vi "PicoScope5000aAdvancedTriggerSettingsV2.vi"(0 "error in":errorcluster, 1 "handle in":i16=16384, 3 "Trigger Conditions":T1 {"Digital Port 1" items=["Don't Care", "True", "False"]; "Digital Port 0" items=["Don't Care", "True", "False"]; "PWQ" items=["Don't Care", "True", "False"]; "Aux" items=["Don't Care", "True", "False"]; "Ext" items=["Don't Care", "True", "False"]; "Channel D" items=["Don't Care", "True", "False"]; "Channel C" items=["Don't Care", "True", "False"]; "Channel B" items=["Don't Care", "True", "False"]; "Channel A" items=["Don't Care", "True", "False"]; "Condition Logic" items=["AND", "OR", "XOR"]}, 4 "Trigger Delay":u32, 5 "Auto Trigger (us)":u64=1000000, 6 "Channel A Trigger Properties":T4={"thresholdUpper"=0, "thresholdUpperHysteresis"=0, "thresholdLower"=0, "thresholdLowerHysteresis"=0, "Threshold Mode"=0, "Direction"=2, "Available"=FALSE} {"Direction" items=["Above / Inside", "Below / Outside", "Rising / Enter", "Falling / Exit", "Rising or Falling / Enter or Exit", "Above Lower", "Below Lower", "Rising Lower", "Falling Lower", "Positive Runt", "Negative Runt"]; "Threshold Mode" items=["Level", "Window"]}, 7 "Channel D Trigger Properties":T4={"thresholdUpper"=0, "thresholdUpperHysteresis"=0, "thresholdLower"=0, "thresholdLowerHysteresis"=0, "Threshold Mode"=0, "Direction"=2, "Available"=FALSE} {"Direction" items=["Above / Inside", "Below / Outside", "Rising / Enter", "Falling / Exit", "Rising or Falling / Enter or Exit", "Above Lower", "Below Lower", "Rising Lower", "Falling Lower", "Positive Runt", "Negative Runt"]; "Threshold Mode" items=["Level", "Window"]}, 8 "Channel B Trigger Properties":T4={"thresholdUpper"=0, "thresholdUpperHysteresis"=0, "thresholdLower"=0, "thresholdLowerHysteresis"=0, "Threshold Mode"=0, "Direction"=2, "Available"=FALSE} {"Direction" items=["Above / Inside", "Below / Outside", "Rising / Enter", "Falling / Exit", "Rising or Falling / Enter or Exit", "Above Lower", "Below Lower", "Rising Lower", "Falling Lower", "Positive Runt", "Negative Runt"]; "Threshold Mode" items=["Level", "Window"]}, 10 "Digital Port  0":T3 {"Direction Channel 7" items=["Don't Care", "Low", "High", "Rising", "Falling"]; "Direction Channel 6" items=["Don't Care", "Low", "High", "Rising", "Falling"]; "Direction Channel 5" items=["Don't Care", "Low", "High", "Rising", "Falling"]; "Direction Channel 4" items=["Don't Care", "Low", "High", "Rising", "Falling"]; "Direction Channel 3" items=["Don't Care", "Low", "High", "Rising", "Falling"]; "Direction Channel 2" items=["Don't Care", "Low", "High", "Rising", "Falling"]; "Direction Channel 1" items=["Don't Care", "Low", "High", "Rising", "Falling"]; "Direction Channel 0" items=["Don't Care", "Low", "High", "Rising", "Falling"]}, 11 "Ext. Trigger Properties":T4={"thresholdUpper"=0, "thresholdUpperHysteresis"=0, "thresholdLower"=0, "thresholdLowerHysteresis"=0, "Threshold Mode"=0, "Direction"=2, "Available"=FALSE} {"Direction" items=["Above / Inside", "Below / Outside", "Rising / Enter", "Falling / Exit", "Rising or Falling / Enter or Exit", "Above Lower", "Below Lower", "Rising Lower", "Falling Lower", "Positive Runt", "Negative Runt"]; "Threshold Mode" items=["Level", "Window"]}, 12 "Digital Port  1":T2 {"Direction Channel 15" items=["Don't Care", "Low", "High", "Rising", "Falling"]; "Direction Channel 14" items=["Don't Care", "Low", "High", "Rising", "Falling"]; "Direction Channel 13" items=["Don't Care", "Low", "High", "Rising", "Falling"]; "Direction Channel 12" items=["Don't Care", "Low", "High", "Rising", "Falling"]; "Direction Channel 11" items=["Don't Care", "Low", "High", "Rising", "Falling"]; "Direction Channel 10" items=["Don't Care", "Low", "High", "Rising", "Falling"]; "Direction Channel 9" items=["Don't Care", "Low", "High", "Rising", "Falling"]; "Direction Channel 8" items=["Don't Care", "Low", "High", "Rising", "Falling"]}, 13 "Aux. Trigger Properties (DO NOT USE)":T4={"thresholdUpper"=0, "thresholdUpperHysteresis"=0, "thresholdLower"=0, "thresholdLowerHysteresis"=0, "Threshold Mode"=0, "Direction"=2, "Available"=FALSE} {"Direction" items=["Above / Inside", "Below / Outside", "Rising / Enter", "Falling / Exit", "Rising or Falling / Enter or Exit", "Above Lower", "Below Lower", "Rising Lower", "Falling Lower", "Positive Runt", "Negative Runt"]; "Threshold Mode" items=["Level", "Window"]}, 16 "Channel C Trigger Properties":T4={"thresholdUpper"=0, "thresholdUpperHysteresis"=0, "thresholdLower"=0, "thresholdLowerHysteresis"=0, "Threshold Mode"=0, "Direction"=2, "Available"=FALSE} {"Direction" items=["Above / Inside", "Below / Outside", "Rising / Enter", "Falling / Exit", "Rising or Falling / Enter or Exit", "Above Lower", "Below Lower", "Rising Lower", "Falling Lower", "Positive Runt", "Negative Runt"]; "Threshold Mode" items=["Level", "Window"]}, 18 "Pulse Width Qualifier Conditions":T6 {"Condition Logic" items=["AND", "OR", "XOR"]}, 19 "Pulse Width Qualifier Settings":T5={"Direction"=2, "Lower Limit"=0, "Upper Limit"=0, "Pulse Width Type"=0} {"Pulse Width Type" items=["None", "Less Than", "Greater Than", "In Range", "Out of Range"]; "Direction" items=["Rising"=2, "Falling"=3, "Rising Lower"=7, "Above"=0, "Below"=1, "Rising or Falling"=4, "Falling Lower"=8, "Below Lower"=6, "Above Lower"=5]}) -> (14 "error out":errorcluster, 15 "handle out":i16=16384)   [LabVIEW 2010]
doc: "This VI is an interface for the advanced trigger features of the oscilloscope (Using V2 functions now recommended)\nA simple trigger can be set using PicoScope5000aSettings.vi, in which case it is not necessary to use this VI."
uses:
  ps5000a.dll
panel:
  out "XOR Debug Array":u32[][](array[numeric])
  in  "SetTrigger Info Action XOR":bool=TRUE
  in  "SetTrigger Info Action OR":bool=TRUE
  # "For Condition Logic Suggested settings;\nFor AND, XOR logic-(parallel triggers)\nUse level-type triggers (Level or Inside/outside Window Triggers)\n\nFor OR logic- (single channel)\nUse edge types (e.g. rising, falling, entering window)"
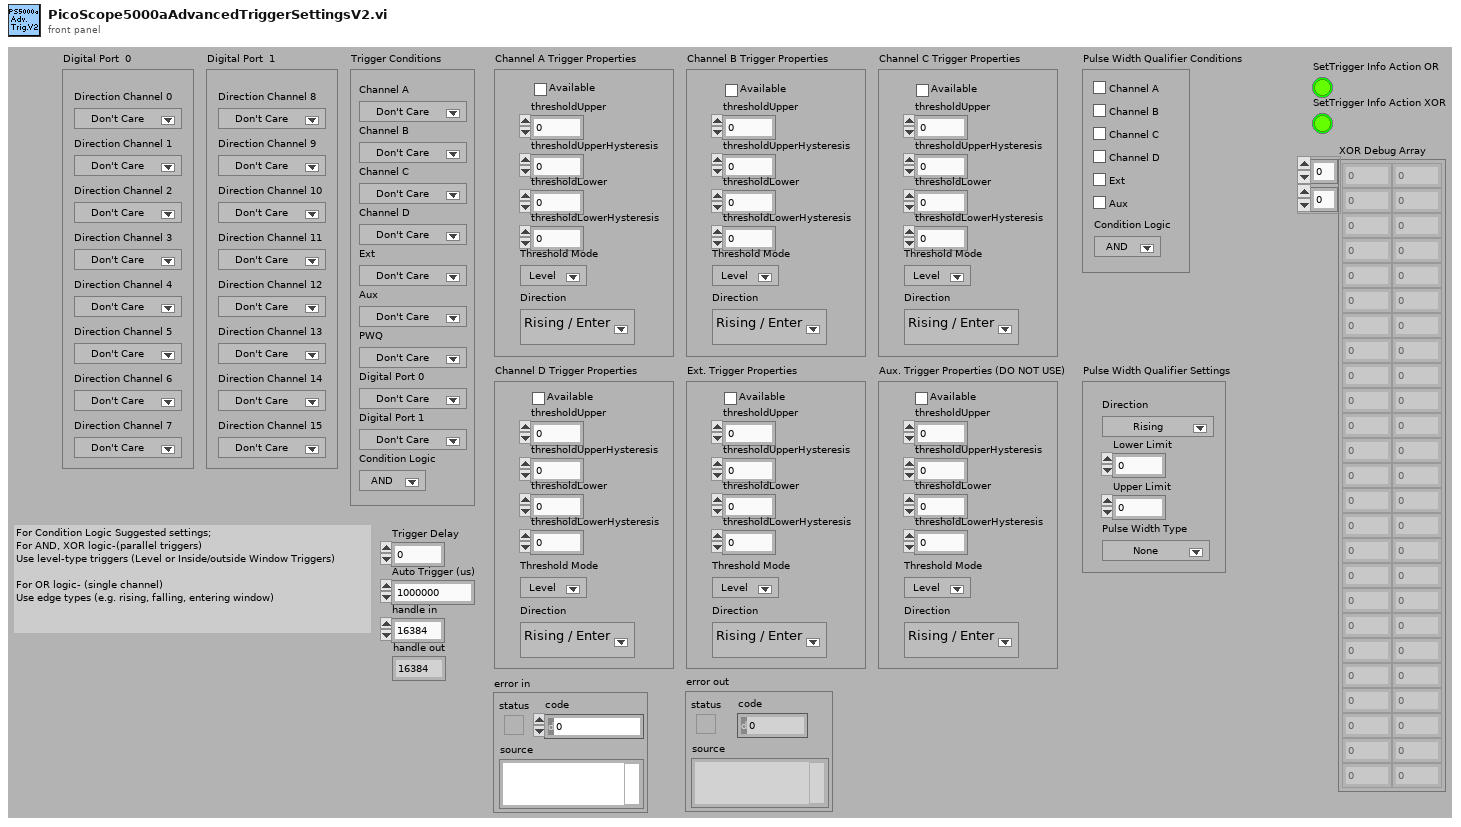
[diagram p1: front panel]
types:
  T1 = cluster{"Channel A":u16, "Channel B":u16, "Channel C":u16, "Channel D":u16, "Ext":u16, "Aux":u16, "PWQ":u16, "Digital Port 0":u16, "Digital Port 1":u16, "Condition Logic":u16}
  T2 = cluster{"Direction Channel 8":u16, "Direction Channel 9":u16, "Direction Channel 10":u16, "Direction Channel 11":u16, "Direction Channel 12":u16, "Direction Channel 13":u16, "Direction Channel 14":u16, "Direction Channel 15":u16}
  T3 = cluster{"Direction Channel 0":u16, "Direction Channel 1":u16, "Direction Channel 2":u16, "Direction Channel 3":u16, "Direction Channel 4":u16, "Direction Channel 5":u16, "Direction Channel 6":u16, "Direction Channel 7":u16}
  T4 = cluster{"thresholdUpper":i16, "thresholdUpperHysteresis":u16, "thresholdLower":i16, "thresholdLowerHysteresis":u16, "Threshold Mode":i32, "Direction":i32, "Available":bool}
  T5 = cluster{"Direction":u32, "Lower Limit":u32, "Upper Limit":u32, "Pulse Width Type":u32}
  T6 = cluster{"Channel A":bool, "Channel B":bool, "Channel C":bool, "Channel D":bool, "Aux":bool, "Condition Logic":u16, "Ext":bool}
  T7 = cluster{"status":bool, "code":u32, "source":string}
  T8 = cluster{"thresholdUpper":i16, "thresholdUpperHysteresis":u16, "thresholdLower":i16, "thresholdLowerHysteresis":u16, "Threshold Mode":i32, "Direction":i32, "Available":bool}[]
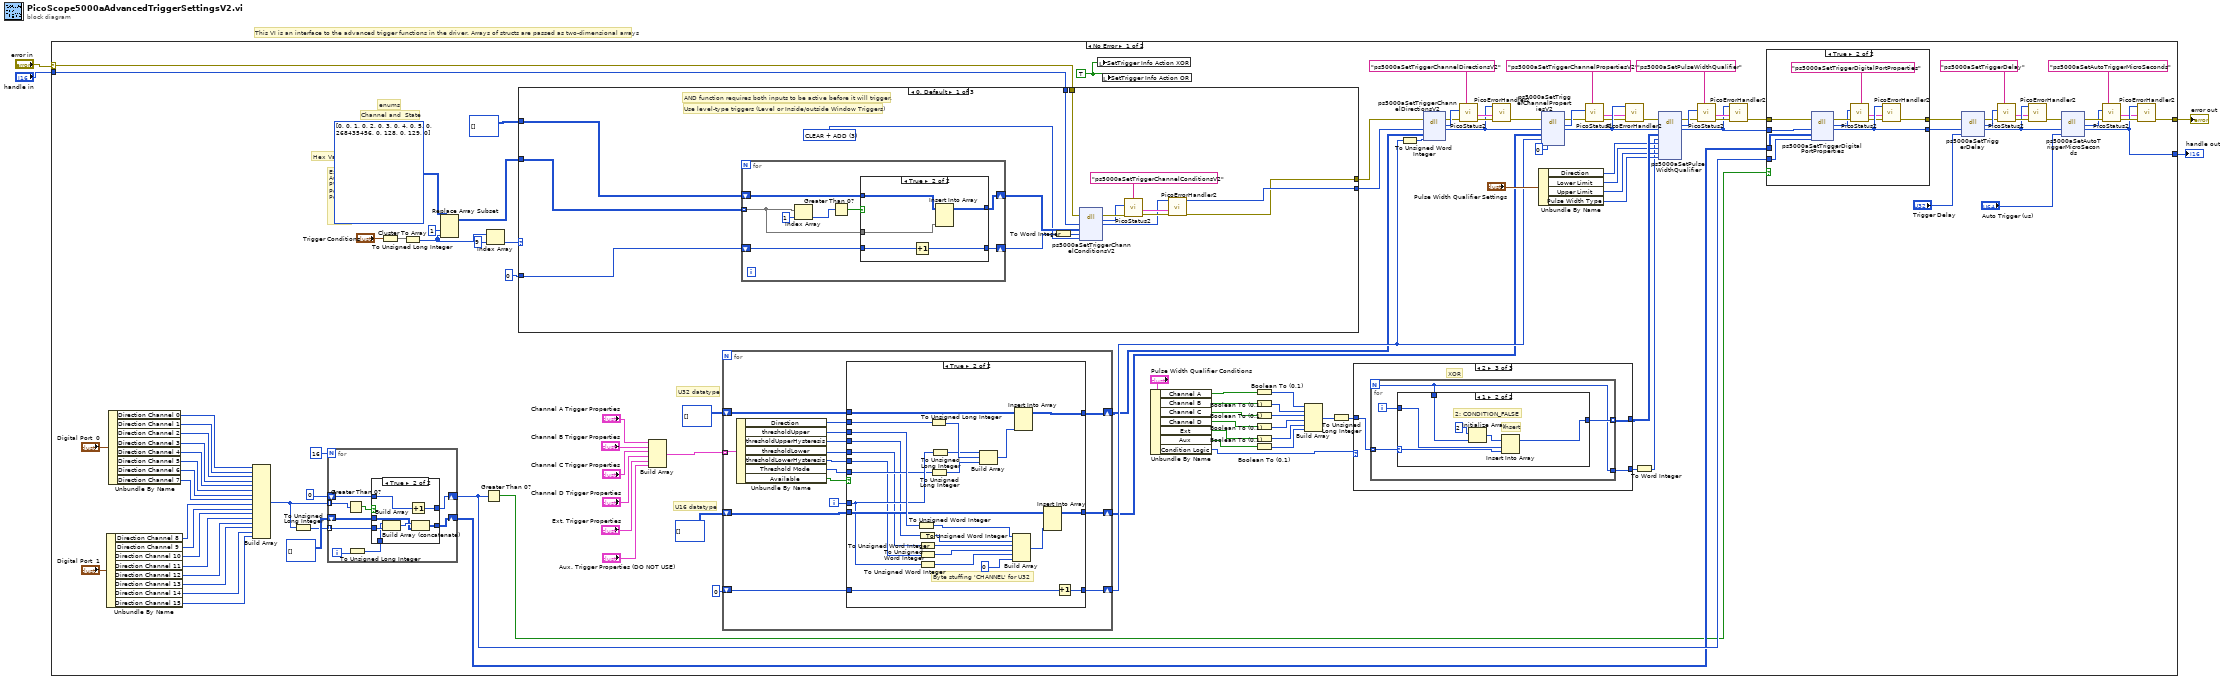
[diagram p0: block diagram]
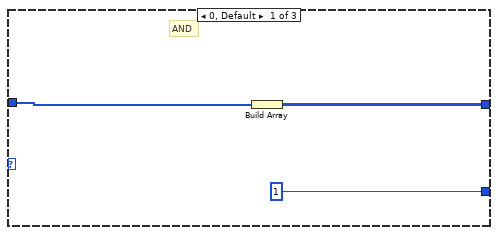
[diagram p4: hidden frame]
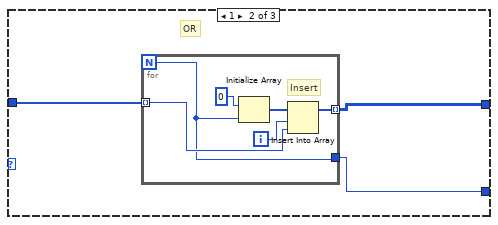
[diagram p5: hidden frame]
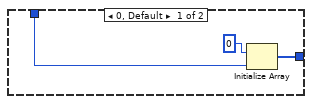
[diagram p6: hidden frame]
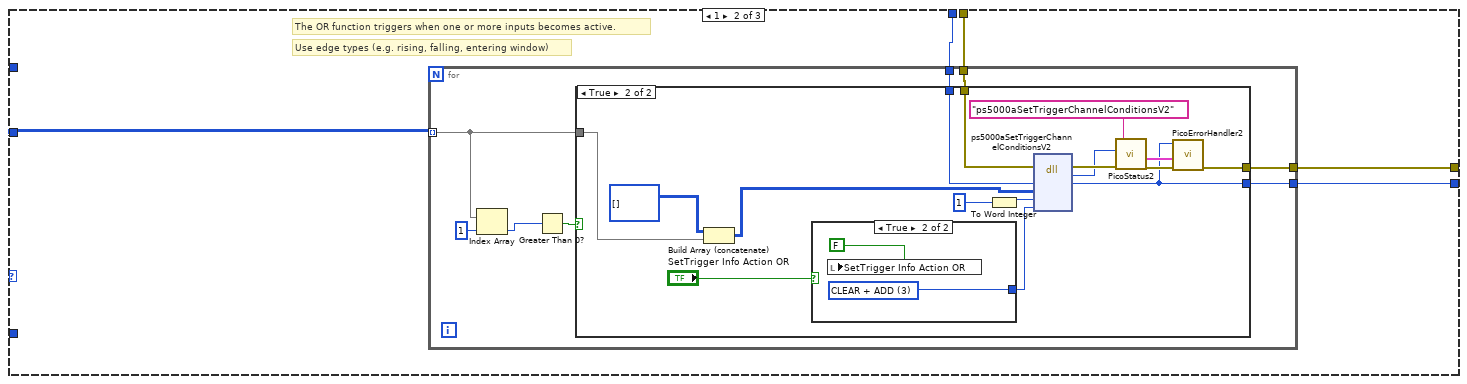
[diagram p9: hidden frame]
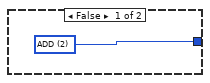
[diagram p11: hidden frame]
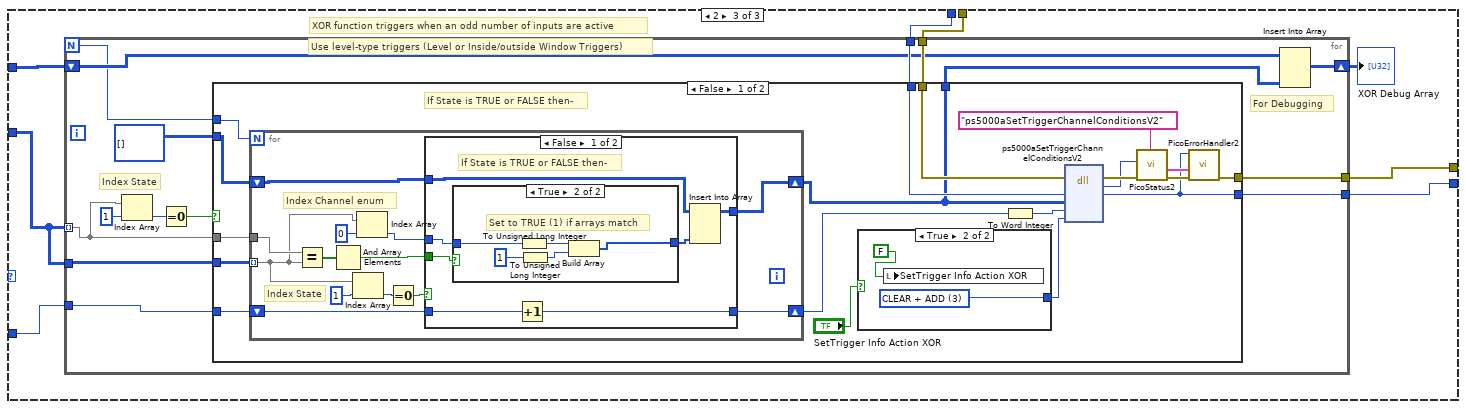
[diagram p12: hidden frame]
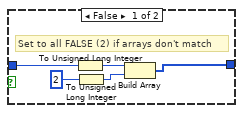
[diagram p13: hidden frame]
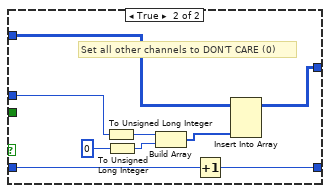
[diagram p14: hidden frame]
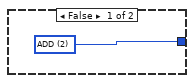
[diagram p15: hidden frame]
diagram:
  # "This VI is an interface to the advanced trigger functions in the driver. Arrays of structs are passed as two-dimensional arrays"
  n1 = case shown="No Error" "error in" {
    selector: "error in" -> [w60 w377]
    tunnel: "handle in" -> [w59 w378]
    tunnel: [w47 w378] -> w2
    tunnel: [w48 w377] -> w1
    frame No Error {
      w53 = TRUE ("Boolean")
      # "enums"
      # "Ext\nAux\nPWQ\nPort0\nPort1"
      # "Channel and  State"
      # "Hex Values"
      # "U16 datatype"
      # "U32 datatype"
      n2 = Unbundle By Name("Digital Port  1") -> ("Direction Channel 8"=w83:u16, "Direction Channel 9"=w82:u16, "Direction Channel 10"=w81:u16, "Direction Channel 11"=w80:u16, "Direction Channel 12"=w79:u16, "Direction Channel 13"=w78:u16, "Direction Channel 14"=w77:u16, "Direction Channel 15"=w76:u16)
      n3 = Unbundle By Name("Digital Port  0") -> ("Direction Channel 0"=w75:u16, "Direction Channel 1"=w92:u16, "Direction Channel 2"=w91:u16, "Direction Channel 3"=w90:u16, "Direction Channel 4"=w89:u16, "Direction Channel 5"=w88:u16, "Direction Channel 6"=w87:u16, "Direction Channel 7"=w86:u16)
      n4 = Build Array(w75, w92, w91, w90, w89, w88, w87, w86, w83, w82, w81, w80, w79, w78, w77, w76) -> (w66:u16[])
      n5 = To Unsigned Long Integer(number=w66) -> (unsigned 32bit integer=w67:u32[])
      n6 = for {
        N: 16 -> [_]
        tunnel: w67 -> [w143] mode=indexing
        shift-right: [w144] -> w71
        shift-left: i16 0 -> [w145]
        shift-right: [w141] -> w70
        shift-left: u32[][] [] -> [w142]
        tunnel: w66 -> [w139] mode=indexing
        i -> [w138]
        n7 = Greater Than 0?(x=w139) -> (x > 0?=w140:bool)
        n8 = To Unsigned Long Integer(number=w138) -> (unsigned 32bit integer=w137:u32)
        n9 = case shown="True" w140 {
          tunnel: w145 -> [w147 w154]
          tunnel: [w147 w151] -> w144
          tunnel: w143 -> [_ w153]
          tunnel: w137 -> [_ w152]
          tunnel: w142 -> [w146 w149]
          tunnel: [w146 w148] -> w141
          frame False {
          }
          frame True {
            n10 = Build Array(w152, w153) -> (w150:u32[])
            n11 = Increment(x=w154) -> (x+1=w151:i16)
            n12 = Build Array (concatenate)(w150, w149) -> (w148:u32[][])
          }
        }
      }
      n13 = Cluster To Array(cluster="Trigger Conditions") -> (array=w42:u16[])
      n14 = To Unsigned Long Integer(number=w42) -> (unsigned 32bit integer=w40:u32[])
      n15 = Replace Array Subset(array=u32[][] [[0, 0], [1, 0], [2, 0], [3, 0], [4, 0], [5, 0], [268435456, 0], [128, 0], [129, 0]], new element=w40, index (col)=1 ("disabled index (col)")) -> (w41:u32[][])  [unwired: 1 in]
      n16 = Greater Than 0?(x=w71) -> (x > 0?=w46:bool)
      n17 = Index Array(array=w40, index=9) -> (element=w38:u32)
      n18 = case shown="0, Default" w38 {
        tunnel: u32[][] [] -> [w240 _ w293]
        tunnel: i16 0 -> [w239 _ w290]
        tunnel: w60 -> [w233 w260 w297]
        tunnel: w59 -> [w232 w259 w296]
        tunnel: [w225 w258 w295] -> w58
        tunnel: [w226 w257 w294] -> w57
        tunnel: w41 -> [w229 w256 w291]
        frame 0, Default {
          w230 = u32 3 items=["CLEAR + ADD"=3, "CLEAR"=1, "ADD"=2] ("Condition Action")
          # "AND function requires both inputs to be active before it will trigger."
          # "Use level-type triggers (Level or Inside/outside Window Triggers)"
          n19 = for {
            shift-right: [w247] -> w235
            shift-left: w239 -> [w246]
            shift-right: [w245] -> w231
            shift-left: w240 -> [w248]
            tunnel: w229 -> [w243] mode=indexing
            n20 = Index Array(array=w243, index=1) -> (element=w242:u32)
            n21 = Greater Than 0?(x=w242) -> (x > 0?=w244:bool)
            n22 = case shown="True" w244 {
              tunnel: w248 -> [w250 w255]
              tunnel: [w250 w254] -> w245
              tunnel: [w249 w253] -> w247
              tunnel: w246 -> [w249 w252]
              tunnel: w243 -> [_ w251]
              frame False {
              }
              frame True {
                n23 = Increment(x=w252) -> (x+1=w253:i16)
                n24 = Insert Into Array(array=w255, new element=w251) -> (w254:u32[][])  [unwired: 2 in]
              }
            }
          }
          n25 = To Word Integer(number=w235) -> (16bit integer=w238:i16)
          n26 = dll-call lib="ps5000a.dll" fn="ps5000aSetTriggerChannelConditionsV2" ("ps3000.dll:_ps3000_open_unit@0")(error in=w233, "handle"=w232, "conditions"=w231, "nConditions"=w238, "info"=w230) -> (error out=w237:errorcluster, "PICO_STATUS"=w236:u32, "handle"=w226:i16)  [unwired: 5 in, 1 out]
          n27 = call "PicoStatus2.vi"("PICO source"="ps5000aSetTriggerChannelConditionsV2" ("source"), "Error in"=w237, "PICO STATUS"=w236) -> ("error out"=w228:errorcluster, "PICO_STATUS out"=w227:T7)  [unwired: 5 in]
          n28 = call "PicoErrorHandler2.vi"("error in (no error)"=w228, "PICO_STATUS in"=w227, "handle In"=w226) -> ("error out"=w225:errorcluster)  [unwired: 8 in]
        }
        frame 1 {
          # "Use edge types (e.g. rising, falling, entering window)"
          # "The OR function triggers when one or more inputs becomes active."
          n29 = for {
            tunnel: w260 -> [w268]
            tunnel: w259 -> [w267]
            tunnel: [w266] -> w258
            tunnel: [w265] -> w257
            tunnel: w256 -> [w263] mode=indexing
            n30 = Index Array(array=w263, index=1) -> (element=w262:u32)
            n31 = Greater Than 0?(x=w262) -> (x > 0?=w261:bool)
            n32 = case shown="True" w261 {
              tunnel: w268 -> [w269 w282]
              tunnel: w267 -> [w270 w281]
              tunnel: [w269 w271] -> w266
              tunnel: [w270 w272] -> w265
              tunnel: w263 -> [_ w275]
              frame False {
              }
              frame True {
                n33 = Build Array (concatenate)(u32[][] [], w275) -> (w277:u32[][])
                n34 = case shown="True" "SetTrigger Info Action OR" {
                  tunnel: [w287 w289] -> w280
                  frame False {
                    w287 = u32 2 items=["CLEAR"=1, "ADD"=2, "CLEAR + ADD"=3] ("Condition Action")
                  }
                  frame True {
                    w289 = u32 3 items=["CLEAR"=1, "ADD"=2, "CLEAR + ADD"=3] ("Condition Action")
                    n35 = local write "SetTrigger Info Action OR"(FALSE ("Boolean")) -> ()
                  }
                }
                n36 = To Word Integer(number=i16 1) -> (16bit integer=w286:i16)
                n37 = dll-call lib="ps5000a.dll" fn="ps5000aSetTriggerChannelConditionsV2" ("ps3000.dll:_ps3000_open_unit@0")(error in=w282, "handle"=w281, "conditions"=w277, "nConditions"=w286, "info"=w280) -> (error out=w285:errorcluster, "PICO_STATUS"=w284:u32, "handle"=w272:i16)  [unwired: 5 in, 1 out]
                n38 = call "PicoStatus2.vi"("PICO source"="ps5000aSetTriggerChannelConditionsV2" ("source"), "Error in"=w285, "PICO STATUS"=w284) -> ("error out"=w274:errorcluster, "PICO_STATUS out"=w273:T7)  [unwired: 5 in]
                n39 = call "PicoErrorHandler2.vi"("error in (no error)"=w274, "PICO_STATUS in"=w273, "handle In"=w272) -> ("error out"=w271:errorcluster)  [unwired: 8 in]
              }
            }
          }
        }
        frame 2 {
          # "Use level-type triggers (Level or Inside/outside Window Triggers)"
          # "XOR function triggers when an odd number of inputs are active"
          n40 = for {
            N -> [w305]
            tunnel: w297 -> [w312]
            tunnel: w296 -> [w311]
            tunnel: [w310] -> w295
            tunnel: [w309] -> w294
            shift-right: [w307] -> w292
            shift-left: w293 -> [w308]
            tunnel: w291 -> [w299] mode=indexing
            tunnel: w291 -> [w302]
            tunnel: w290 -> [w303]
            # "Index State"
            # "For Debugging"
            n41 = Index Array(array=w299, index=1) -> (element=w300:u32)
            n42 = Equal To 0?(x=w300) -> (x = 0?=w298:bool)
            n43 = case shown="False" w298 {
              tunnel: w312 -> [w331 w374]
              tunnel: w311 -> [w330 w375]
              tunnel: [w316 w374] -> w310
              tunnel: [w313 w375] -> w309
              tunnel: [w328 w376] -> w306
              tunnel: w305 -> [w327 _]
              tunnel: u32[][] [] -> [w326 w376]
              tunnel: w303 -> [w325 _]
              tunnel: w302 -> [w324 _]
              tunnel: w299 -> [w323 _]
              frame False {
                # "If State is TRUE or FALSE then-"
                n44 = for {
                  N: w327 -> [_]
                  shift-right: [w343] -> w329
                  shift-left: w325 -> [w344]
                  shift-right: [w332] -> w328
                  shift-left: w326 -> [w333]
                  tunnel: w323 -> [w340]
                  tunnel: w324 -> [w336] mode=indexing
                  # "Index State"
                  # "Index Channel enum"
                  n45 = Equal?(x=w340, y=w336) -> (x = y?=w334:bool[])
                  n46 = And Array Elements(Boolean array=w334) -> (logical AND=w339:bool)
                  n47 = Index Array(array=w336, index=1) -> (element=w337:u32)
                  n48 = Index Array(array=w336, index=0) -> (element=w341:u32)
                  n49 = Equal To 0?(x=w337) -> (x = 0?=w335:bool)
                  n50 = case shown="False" w335 {
                    tunnel: w344 -> [w351 w362]
                    tunnel: [w350 w363] -> w343
                    tunnel: w341 -> [w349 w366]
                    tunnel: w339 -> [w348 _]
                    tunnel: w333 -> [w347 w365]
                    tunnel: [w345 w364] -> w332
                    frame False {
                      # "If State is TRUE or FALSE then-"
                      n51 = case shown="True" w348 {
                        tunnel: [w356 w361] -> w346
                        tunnel: w349 -> [w355 w360]
                        frame False {
                          # "Set to all FALSE (2) if arrays don't match"
                          n52 = To Unsigned Long Integer(number=w355) -> (unsigned 32bit integer=w353:u32)
                          n53 = To Unsigned Long Integer(number=u32 2) -> (unsigned 32bit integer=w354:u32)
                          n54 = Build Array(w353, w354) -> (w356:u32[])
                        }
                        frame True {
                          # "Set to TRUE (1) if arrays match"
                          n55 = To Unsigned Long Integer(number=w360) -> (unsigned 32bit integer=w358:u32)
                          n56 = To Unsigned Long Integer(number=u32 1) -> (unsigned 32bit integer=w359:u32)
                          n57 = Build Array(w358, w359) -> (w361:u32[])
                        }
                      }
                      n58 = Increment(x=w351) -> (x+1=w350:i16)
                      n59 = Insert Into Array(array=w347, new element=w346) -> (w345:u32[][])  [unwired: 2 in]
                    }
                    frame True {
                      # "Set all other channels to DON'T CARE (0)"
                      n60 = To Unsigned Long Integer(number=w366) -> (unsigned 32bit integer=w368:u32)
                      n61 = To Unsigned Long Integer(number=u32 0) -> (unsigned 32bit integer=w369:u32)
                      n62 = Build Array(w368, w369) -> (w370:u32[])
                      n63 = Increment(x=w362) -> (x+1=w363:i16)
                      n64 = Insert Into Array(array=w365, new element=w370) -> (w364:u32[][])  [unwired: 2 in]
                    }
                  }
                }
                n65 = case shown="True" "SetTrigger Info Action XOR" {
                  tunnel: [w371 w373] -> w318
                  frame False {
                    w371 = u32 2 items=["CLEAR + ADD"=3, "CLEAR"=1, "ADD"=2] ("Condition Action")
                  }
                  frame True {
                    w373 = u32 3 items=["CLEAR + ADD"=3, "CLEAR"=1, "ADD"=2] ("Condition Action")
                    n66 = local write "SetTrigger Info Action XOR"(FALSE ("Boolean")) -> ()
                  }
                }
                n67 = To Word Integer(number=w329) -> (16bit integer=w322:i16)
                n68 = dll-call lib="ps5000a.dll" fn="ps5000aSetTriggerChannelConditionsV2" ("ps3000.dll:_ps3000_open_unit@0")(error in=w331, "handle"=w330, "conditions"=w328, "nConditions"=w322, "info"=w318) -> (error out=w321:errorcluster, "PICO_STATUS"=w317:u32, "handle"=w313:i16)  [unwired: 5 in, 1 out]
                n69 = call "PicoStatus2.vi"("PICO source"="ps5000aSetTriggerChannelConditionsV2" ("source"), "Error in"=w321, "PICO STATUS"=w317) -> ("error out"=w315:errorcluster, "PICO_STATUS out"=w314:T7)  [unwired: 5 in]
                n70 = call "PicoErrorHandler2.vi"("error in (no error)"=w315, "PICO_STATUS in"=w314, "handle In"=w313) -> ("error out"=w316:errorcluster)  [unwired: 8 in]
              }
              frame True {
              }
            }
            n71 = Insert Into Array(array=w308, new element=w306) -> (w307:u32[][])  [unwired: 2 in]
          }
          "XOR Debug Array" <- w292
        }
      }
      n72 = Build Array("Channel A Trigger Properties", "Channel B Trigger Properties", "Channel C Trigger Properties", "Channel D Trigger Properties", "Ext. Trigger Properties", "Aux. Trigger Properties (DO NOT USE)") -> (w121:T8)
      n73 = for {
        tunnel: w121 -> [w192] mode=indexing
        shift-right: [w189] -> w63
        shift-left: i16 0 -> [w188]
        shift-right: [w186] -> w36
        shift-left: u16[][] [] -> [w187]
        shift-right: [w185] -> w37
        shift-left: u32[][] [] -> [w184]
        i -> [w190]
        n74 = Unbundle By Name(w192) -> ("Direction"=w183:i32, "thresholdUpper"=w197:i16, "thresholdUpperHysteresis"=w196:u16, "thresholdLower"=w195:i16, "thresholdLowerHysteresis"=w194:u16, "Threshold Mode"=w193:i32, "Available"=w191:bool)
        n75 = case shown="True" w191 {
          tunnel: w197 -> [_ w224]
          tunnel: w196 -> [_ w204]
          tunnel: w195 -> [_ w203]
          tunnel: w194 -> [_ w202]
          tunnel: w193 -> [_ w212]
          tunnel: w190 -> [_ w214]
          tunnel: [w200 w222] -> w189
          tunnel: w188 -> [w200 w221]
          tunnel: [w199 w219] -> w186
          tunnel: w187 -> [w199 w218]
          tunnel: [w198 w217] -> w185
          tunnel: w184 -> [w198 w216]
          tunnel: w183 -> [_ w213]
          frame False {
          }
          frame True {
            # "Byte stuffing 'CHANNEL' for U32"
            n76 = To Unsigned Word Integer(number=w224) -> (unsigned 16bit integer=w206:u16)
            n77 = To Unsigned Word Integer(number=w204) -> (unsigned 16bit integer=w205:u16)
            n78 = To Unsigned Word Integer(number=w203) -> (unsigned 16bit integer=w201:u16)
            n79 = To Unsigned Word Integer(number=w202) -> (unsigned 16bit integer=w207:u16)
            n80 = To Unsigned Word Integer(number=w214) -> (unsigned 16bit integer=w208:u16)
            n81 = To Unsigned Long Integer(number=w213) -> (unsigned 32bit integer=w210:u32)
            n82 = To Unsigned Long Integer(number=w212) -> (unsigned 32bit integer=w211:u32)
            n83 = To Unsigned Long Integer(number=w214) -> (unsigned 32bit integer=w209:u32)
            n84 = Build Array(w209, w210, w211) -> (w215:u32[])
            n85 = Build Array(w206, w205, w201, w207, w208, u16 0 ("element")) -> (w220:u16[])
            n86 = Insert Into Array(array=w216, new element=w215) -> (w217:u32[][])  [unwired: 2 in]
            n87 = Insert Into Array(array=w218, new element=w220) -> (w219:u16[][])  [unwired: 2 in]
            n88 = Increment(x=w221) -> (x+1=w222:i16)
          }
        }
      }
      n89 = local write "SetTrigger Info Action XOR"(w53) -> ()
      n90 = local write "SetTrigger Info Action OR"(w53) -> ()
      n91 = Unbundle By Name("Pulse Width Qualifier Conditions") -> ("Channel A"=w28:bool, "Channel B"=w27:bool, "Channel C"=w26:bool, "Channel D"=w25:bool, "Ext"=w24:bool, "Aux"=w23:bool, "Condition Logic"=w21:u16)
      n92 = Boolean To (0,1)(Boolean=w28) -> (0, 1=w31:i16)
      n93 = Boolean To (0,1)(Boolean=w27) -> (0, 1=w32:i16)
      n94 = Boolean To (0,1)(Boolean=w26) -> (0, 1=w33:i16)
      n95 = Boolean To (0,1)(Boolean=w25) -> (0, 1=w34:i16)
      n96 = Boolean To (0,1)(Boolean=w24) -> (0, 1=w35:i16)
      n97 = Boolean To (0,1)(Boolean=w23) -> (0, 1=w30:i16)
      n98 = Build Array(w31, w32, w33, w34, w35, w30) -> (w29:i16[])
      n99 = To Unsigned Long Integer(number=w29) -> (unsigned 32bit integer=w22:u32[])
      n100 = case shown="2" w21 {
        tunnel: [w157 w160 w169] -> w119
        tunnel: [u32 1 w158 w168] -> w20
        tunnel: w22 -> [w155 w159 w167]
        frame 0, Default {
          # "AND"
          n101 = Build Array(w155) -> (w157:u32[][])
        }
        frame 1 {
          # "OR"
          n102 = for {
            N -> [w161]
            tunnel: w159 -> [w163] mode=indexing
            tunnel: [w162] -> w160 mode=indexing
            tunnel: [w161] -> w158
            i -> [w164]
            # "Insert"
            n103 = Initialize Array(u32 0 ("element"), w161) -> (w165:u32[])
            n104 = Insert Into Array(array=w165, index=w164, new element=w163) -> (w162:u32[])
          }
        }
        frame 2 {
          # "XOR"
          n105 = for {
            N -> [w170]
            tunnel: w167 -> [w173] mode=indexing
            tunnel: [w171] -> w169 mode=indexing
            tunnel: [w170] -> w168
            i -> [w172]
            n106 = case shown="1" w173 {
              selector: w173 -> [_ w179]
              tunnel: [w175 w180] -> w171
              tunnel: w172 -> [_ w178]
              tunnel: w170 -> [w174 w177]
              frame 0, Default {
                n107 = Initialize Array(u32 0 ("element"), w174) -> (w175:u32[])
              }
              frame 1 {
                # "2: CONDITION_FALSE"
                # "Insert"
                n108 = Initialize Array(u32 2 ("element"), w177) -> (w181:u32[])
                n109 = Insert Into Array(array=w181, index=w178, new element=w179) -> (w180:u32[])
              }
            }
          }
        }
      }
      n110 = To Unsigned Word Integer(number=w63) -> (unsigned 16bit integer=w64:u16)
      n111 = dll-call lib="ps5000a.dll" fn="ps5000aSetTriggerChannelDirectionsV2" ("ps3000.dll:_ps3000_open_unit@0")(error in=w58, "handle"=w57, "directions"=w37, "nDirections"=w64) -> (error out=w107:errorcluster, "PICO_STATUS"=w108:u32, "handle"=w14:i16)  [unwired: 4 in, 1 out]
      n112 = call "PicoStatus2.vi"("PICO source"="ps5000aSetTriggerChannelDirectionsV2" ("source"), "Error in"=w107, "PICO STATUS"=w108) -> ("error out"=w16:errorcluster, "PICO_STATUS out"=w17:T7)  [unwired: 5 in]
      n113 = call "PicoErrorHandler2.vi"("error in (no error)"=w16, "PICO_STATUS in"=w17, "handle In"=w14) -> ("error out"=w13:errorcluster)  [unwired: 8 in]
      n114 = Unbundle By Name("Pulse Width Qualifier Settings") -> ("Direction"=w117:u32, "Lower Limit"=w116:u32, "Upper Limit"=w115:u32, "Pulse Width Type"=w114:u32)
      n115 = dll-call lib="ps5000a.dll" fn="ps5000aSetTriggerChannelPropertiesV2" ("ps3000.dll:_ps3000_open_unit@0")(error in=w13, "handle"=w14, "channelProperties"=w36, "nChannelProperties"=w63, "auxOutputEnable"=i16 0) -> (error out=w105:errorcluster, "PICO_STATUS"=w106:u32, "handle"=w12:i16)  [unwired: 5 in, 1 out]
      n116 = call "PicoStatus2.vi"("PICO source"="ps5000aSetTriggerChannelPropertiesV2" ("source"), "Error in"=w105, "PICO STATUS"=w106) -> ("error out"=w11:errorcluster, "PICO_STATUS out"=w10:T7)  [unwired: 5 in]
      n117 = call "PicoErrorHandler2.vi"("error in (no error)"=w11, "PICO_STATUS in"=w10, "handle In"=w12) -> ("error out"=w9:errorcluster)  [unwired: 8 in]
      n118 = To Word Integer(number=w20) -> (16bit integer=w19:i16)
      n119 = dll-call lib="ps5000a.dll" fn="ps5000aSetPulseWidthQualifier" ("ps3000.dll:_ps3000_open_unit@0")(error in=w9, "handle"=w12, "conditions"=w119, "nConditions"=w19, "direction"=w117, "lower"=w116, "upper"=w115, "type"=w114) -> (error out=w103:errorcluster, "PICO_STATUS"=w104:u32, "handle"=w6:i16)  [unwired: 8 in, 1 out]
      n120 = call "PicoStatus2.vi"("PICO source"="ps5000aSetPulseWidthQualifier" ("source"), "Error in"=w103, "PICO STATUS"=w104) -> ("error out"=w8:errorcluster, "PICO_STATUS out"=w7:T7)  [unwired: 5 in]
      n121 = call "PicoErrorHandler2.vi"("error in (no error)"=w8, "PICO_STATUS in"=w7, "handle In"=w6) -> ("error out"=w15:errorcluster)  [unwired: 8 in]
      n122 = case shown="True" w46 {
        tunnel: w6 -> [w124 w133]
        tunnel: w15 -> [w125 w132]
        tunnel: w71 -> [_ w131]
        tunnel: w70 -> [_ w130]
        tunnel: [w125 w127] -> w69
        tunnel: [w124 w129] -> w68
        frame False {
        }
        frame True {
          n123 = dll-call lib="ps5000a.dll" fn="ps5000aSetTriggerDigitalPortProperties"(error in=w132, "handle"=w133, "digitalDirections"=w130, "nDigitalDirections"=w131) -> (error out=w135:errorcluster, "PICO_STATUS"=w134:u32, "handle"=w129:i16)  [unwired: 4 in, 1 out]
          n124 = call "PicoStatus2.vi"("PICO source"="ps5000aSetTriggerDigitalPortProperties" ("source"), "Error in"=w135, "PICO STATUS"=w134) -> ("error out"=w128:errorcluster, "PICO_STATUS out"=w126:T7)  [unwired: 5 in]
          n125 = call "PicoErrorHandler2.vi"("error in (no error)"=w128, "PICO_STATUS in"=w126, "handle In"=w129) -> ("error out"=w127:errorcluster)  [unwired: 8 in]
        }
      }
      n126 = dll-call lib="ps5000a.dll" fn="ps5000aSetTriggerDelay" ("ps3000.dll:_ps3000_open_unit@0")(error in=w69, "handle"=w68, "delay"="Trigger Delay") -> (error out=w101:errorcluster, "PICO_STATUS"=w102:u32, "handle"=w55:i16)  [unwired: 3 in, 1 out]
      n127 = call "PicoStatus2.vi"("PICO source"="ps5000aSetTriggerDelay" ("source"), "Error in"=w101, "PICO STATUS"=w102) -> ("error out"=w100:errorcluster, "PICO_STATUS out"=w18:T7)  [unwired: 5 in]
      n128 = call "PicoErrorHandler2.vi"("error in (no error)"=w100, "PICO_STATUS in"=w18, "handle In"=w55) -> ("error out"=w56:errorcluster)  [unwired: 8 in]
      n129 = dll-call lib="ps5000a.dll" fn="ps5000aSetAutoTriggerMicroSeconds" ("ps3000.dll:_ps3000_open_unit@0")(error in=w56, "handle"=w55, "autoTriggerMicroseconds"="Auto Trigger (us)") -> (error out=w51:errorcluster, "PICO_STATUS"=w50:u32, "handle"=w47:i16)  [unwired: 3 in, 1 out]
      n130 = call "PicoStatus2.vi"("PICO source"="ps5000aSetAutoTriggerMicroSeconds" ("source"), "Error in"=w51, "PICO STATUS"=w50) -> ("error out"=w52:errorcluster, "PICO_STATUS out"=w5:T7)  [unwired: 5 in]
      n131 = call "PicoErrorHandler2.vi"("error in (no error)"=w52, "PICO_STATUS in"=w5, "handle In"=w47) -> ("error out"=w48:errorcluster)  [unwired: 8 in]
    }
    frame Error {
    }
  }
  "handle out" <- w2
  "error out" <- w1
